vi "OCT Host Emulator.vi"() -> ()   [LabVIEW 2010]
panel:
  out "OCT encoder":dbl
  in  "OCT cmd":dbl step=0.5
  in  "stop":bool
  in  "Translation Array":dbl[](array[numeric])=[0.0, 0.0, 0.0] min=-3.0 max=3.0 step=0.01
  in  "Rotation Array":dbl[](array[numeric])=[0.0, 0.0, 0.0] min=-30.0 max=30.0 step=1.0
  in  "Scaling Array":dbl[](array[numeric])=[1.0, 1.0, 1.0] min=0.5 max=1.5 step=0.05
  # "x scaling"
  # "(mm, negative is down)"
  # "y scaling"
  # "z scaling"
  # "(mm)"
  # "x rotation"
  # "(deg)"
  # "y rotation"
  # "(deg)"
  # "z rotation"
  # "(deg)"
  # "x translation"
  # "(mm)"
  # "y translation"
  # "(mm)"
  # "z translation"
  # "(mm)"
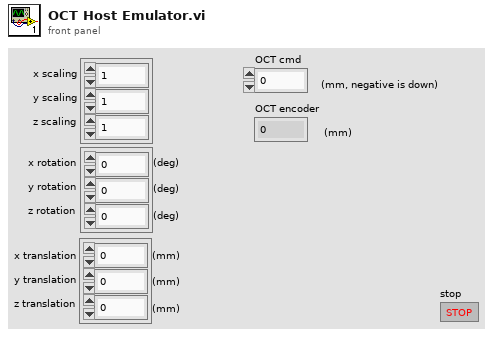
[diagram p1: front panel]
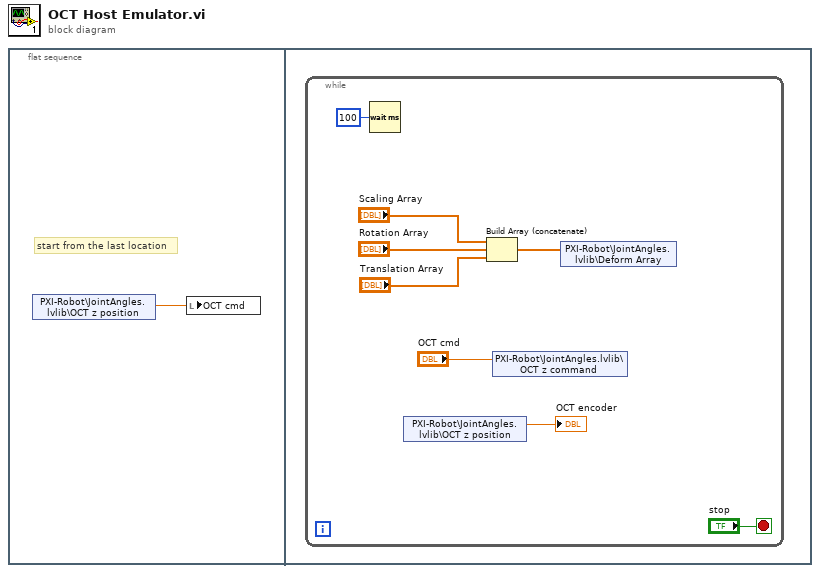
[diagram p0: block diagram]
diagram:
  n1 = flat-sequence {
    frame #0 {
      # "start from the last location"
      n2 = shared-variable "PXI-Robot\\JointAngles.lvlib\\OCT z position"() -> (w1:dbl)  [unwired: 1 in, 1 out]
      n3 = local write "OCT cmd"(w1) -> ()
    }
    frame #1 {
      n4 = while {
        stop <- "stop" stop-if-true
        n5 = Wait (ms)(milliseconds to wait=u32 100) -> ()  [unwired: 1 out]
        n6 = shared-variable "PXI-Robot\\JointAngles.lvlib\\OCT z position"() -> (→"OCT encoder":dbl)  [unwired: 1 in, 1 out]
        n7 = Build Array (concatenate)("Scaling Array", "Rotation Array", "Translation Array") -> (w5:dbl[])
        n8 = shared-variable "PXI-Robot\\JointAngles.lvlib\\OCT z command"("OCT cmd") -> ()  [unwired: 1 in, 1 out]
        n9 = shared-variable "PXI-Robot\\JointAngles.lvlib\\Deform Array"(w5) -> ()  [unwired: 1 in, 1 out]
      }
    }
  }
